vi "Read PumpState.vi"(11 "Pump_1AI_1DO_2DI in":refnum<class "Engine_1DO_2DI.lvclass">) -> (2 "PumpState":T1)   [LabVIEW 2019, in "Engine_1DO_2DI.lvclass"]
uses:
  Engine_1DO_2DI.lvclass
  TypeDef/State Engine.ctl
  Engine_1DO_2DI.lvclass/Engine_1DO_2DI.ctl
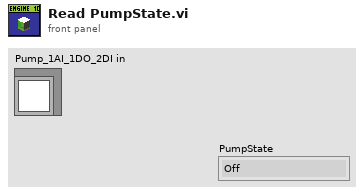
[diagram p1: front panel]
types:
  T1 = typedef "State Engine.ctl" = enum16{"Off", "TupningOn", "On", "TurningOff"}
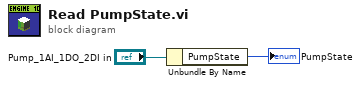
[diagram p0: block diagram]
diagram:
  n1 = Unbundle By Name("Pump_1AI_1DO_2DI in") -> ("PumpState"=→"PumpState":T1)
